vi "Read Sequence Config.lvclass.vi"(8 "error in (no error)":errorcluster, 11 "SequenceNode in":refnum<class "SequenceNode.lvclass">) -> (0 "error out":errorcluster, 2 "Sequence Config.lvclass":refnum<class "Sequence Config.lvclass">, 3 "SequenceNode out":refnum<class "SequenceNode.lvclass">)   [LabVIEW 2015, in "SequenceNode.lvclass"]
uses:
  SequenceNode.lvclass
  Prototype/classes/Sequence/Config/Sequence Config.lvclass
  SequenceNode.lvclass/SequenceNode.ctl
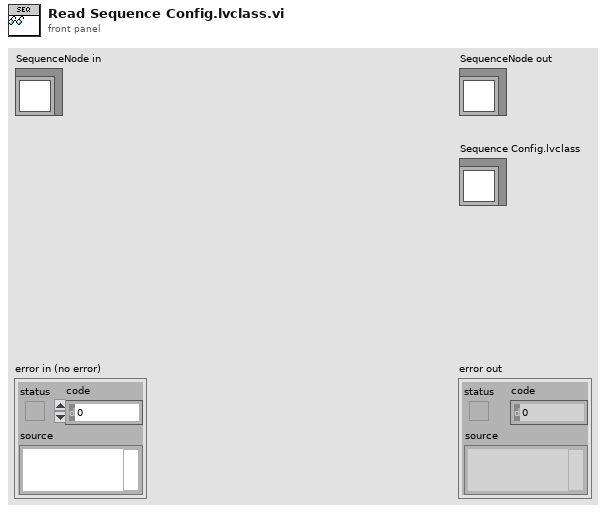
[diagram p1: front panel]
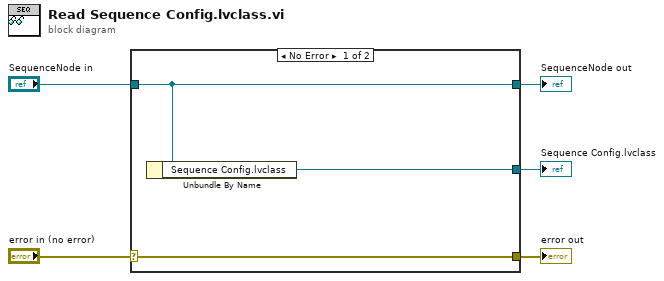
[diagram p0: block diagram]
diagram:
  n1 = case shown="No Error" "error in (no error)" {
    selector: "error in (no error)" -> [w8 w9]
    tunnel: [w8 w9] -> w4
    tunnel: [w7 w10] -> w2
    tunnel: "SequenceNode in" -> [w7 w10]
    tunnel: [w6 _] -> w1
    frame No Error {
      n2 = Unbundle By Name(w7) -> ("Sequence Config.lvclass"=w6:refnum<class "Sequence Config.lvclass">)
    }
    frame Error {
    }
  }
  "error out" <- w4
  "SequenceNode out" <- w2
  "Sequence Config.lvclass" <- w1
